vi "ingresarDatosEquipos.vi"(8 "error in (no error)":errorcluster, 11 "Dosimetro in":refnum<class "Dosimetro.lvclass">) -> (0 "error out":errorcluster, 3 "Dosimetro out":refnum<class "Dosimetro.lvclass">)   [LabVIEW 2019, in "Dosimetro.lvclass"]
uses:
  Dosimetro.lvclass
panel:
  in  "cb_marca_mic 2":string(combo)
  in  "numero_serial_mic 3":string
  in  "numero_serial_mic 2":string
  in  "salir":bool
  in  "numero_serial_mic":string
  in  "cb_marca_mic":string(combo)
  in  "cb_clase_equipo":string(combo)
  out "estandar":string
  in  "cb_cliente":string(combo)
  in  "numero_serial_equipo":string
  out "equipoSeleccionado":string
  in  "cb_marca_equipo":string(combo)
  # "Equipo"
  # "Micrófono"
  # "Cliente"
  # "Dirección"
  # "Nombre"
  # "Número Serial"
  # "Modelo"
  # "Marca"
  # "Clase"
  # "Estándar"
  # "Modelo"
  # "Número Serial"
  # "Marca"
  # "Equipo"
  # "Ingreso Datos de Instrumentos y Accesorios"
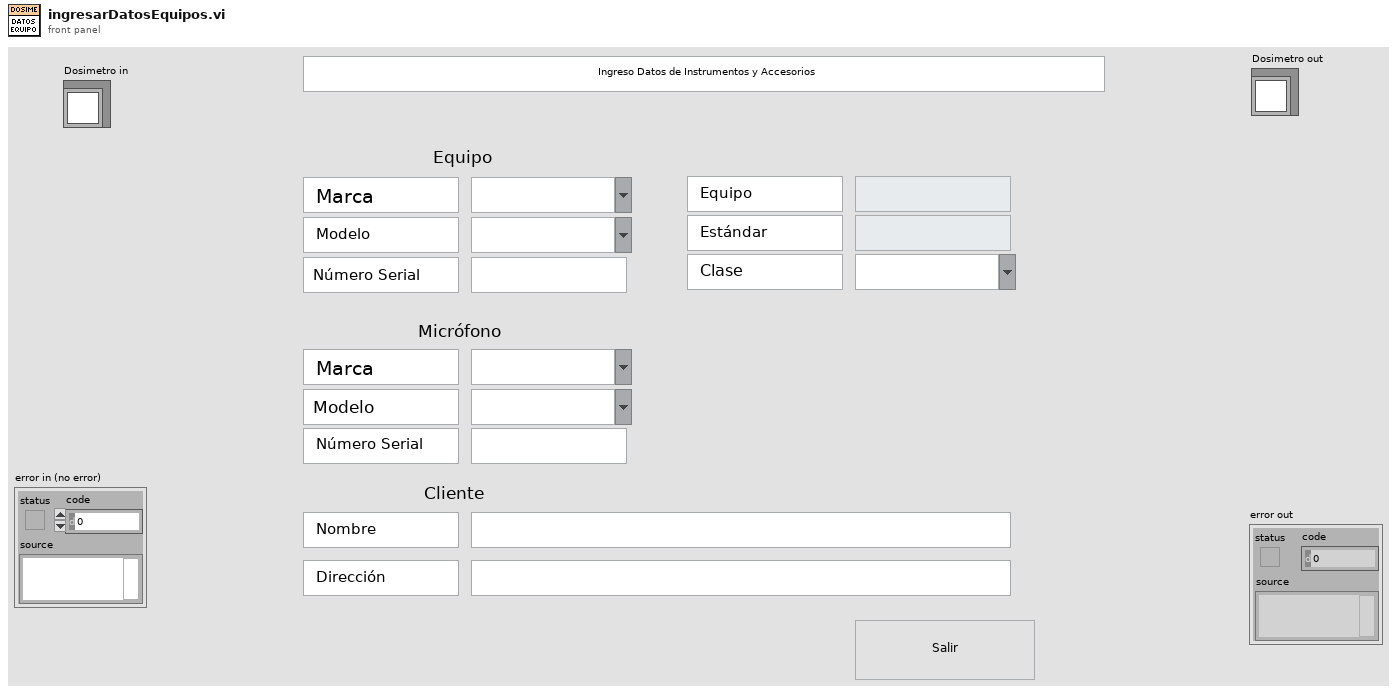
[diagram p1: front panel]
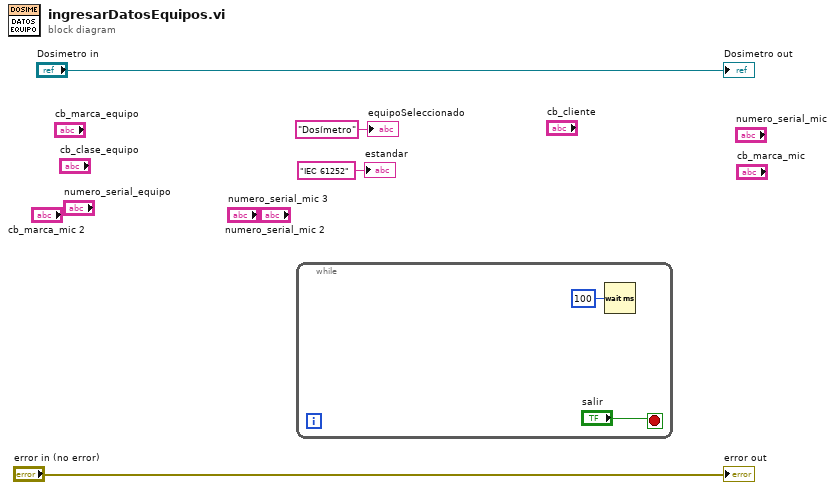
[diagram p0: block diagram]
diagram:
  n1 = while {
    stop <- "salir" stop-if-true
    n2 = Wait (ms)(milliseconds to wait=u32 100) -> ()  [unwired: 1 out]
  }
  "error out" <- "error in (no error)"
  "Dosimetro out" <- "Dosimetro in"
  "equipoSeleccionado" <- "Dosímetro" ("equipoSeleccionado")
  "estandar" <- "IEC 61252" ("estandar")
